vi "AO Write (waveform).vi"(0 "taskID in":u32 format="%x", 5 "waveform data":waveform(dbl)[](array[waveform]), 7 "time limit in sec (no change:-1)":sgl=0.1 format="%0.2f", 9 "allow regeneration (T)":bool=TRUE, 11 "error in (no error)":errorcluster) -> (4 "taskID out":u32 format="%x", 6 "number of updates done":i32, 8 "number of buffers done":i32, 10 "generation complete":bool, 15 "error out":errorcluster)   [LabVIEW 2009]
doc: "Writes data into the buffer for a buffered analog output operation."
uses:
  AO Buffer Write (waveform).vi
panel:
  # "channel\nindex"
  # "Note: t0 and dt are not used by Analog Output"
  # "allow regeneration: T"
  # "no regeneration: F"
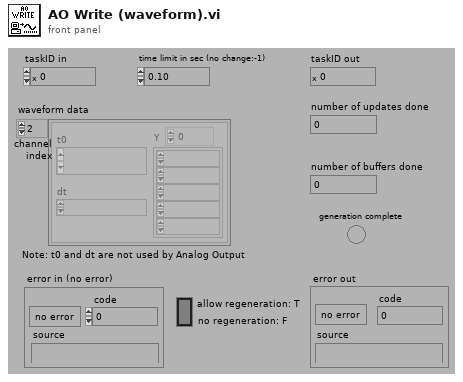
[diagram p1: front panel]
types:
  T1 = enum16{"no change", "relative to write mark", "relative to start of buffer"}
  T2 = enum16{"no such buffer", "active", "finished", "waiting for data", "ready"}
  T3 = enum16{"no change", "allow regeneration ", "do not allow regeneration", "stop after one generation"}
  T4 = cluster{"Cluster Element":i16[][], i32, u32, i32, "write mode":enum16{"no change", "relative to write mark", "relative to start of buffer"}}
  T5 = cluster{"buffer  number":i32, "output mark":i32, "write mark":i32, "buffer iterations":i32, "buffer  state":enum16{"no such buffer", "active", "finished", "waiting for data", "ready"}, "channel state":enum16{"clear", "running", "finished", "paused"}[]}
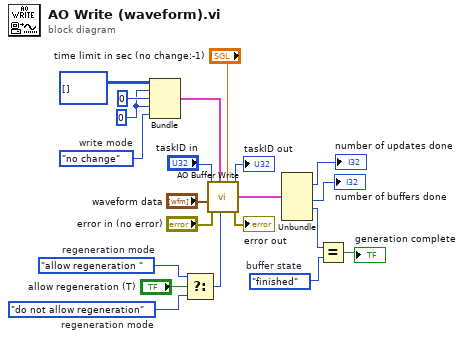
[diagram p0: block diagram]
diagram:
  w4 = T1."no change"  # write mode
  w5 = T2."finished"  # buffer state
  w6 = T3."do not allow regeneration"  # regeneration mode
  w7 = T3."allow regeneration "  # regeneration mode
  w2 = 0
  n1 = Bundle("Cluster Element"=i16[][] [], w2, u32 0, w2, "write mode"=w4) -> (w19:T4)  [unwired: 1 in]
  n2 = Select(t=w7, s="allow regeneration (T)", f=w6) -> (s? t:f=w13:T3)
  n3 = call-poly "AO Buffer Write.vi"("time limit\n(-1: auto calculate)"="time limit in sec (no change:-1)", "regeneration mode (0: no change)"=w13, "alternate data and mode set (no change)"=w19, "error in (no error)"="error in (no error)", "waveform data (empty)"="waveform data", "task ID"="taskID in") -> ("error out"=→"error out":errorcluster, "update progress"=w15:T5, "task ID out"=→"taskID out":u32)  [unwired: 3 in]
  n4 = Unbundle(w15) -> ("output mark"=→"number of updates done":i32, "buffer iterations"=→"number of buffers done":i32, "buffer  state"=w17:T2)  [unwired: 3 out]
  n5 = Equal?(x=w17, y=w5) -> (x = y?=→"generation complete":bool)
